vi "setNSteps.vi"(0 "connection ID":refnum<k5>, 1 "axis":i32, 2 "backward":bool, 3 "step":i32, 5 "error in":errorcluster) -> (14 "connection ID":refnum<k5>, 15 "axis_out":i32, 19 "error out":errorcluster)   [LabVIEW 2016]
doc: "This function triggers n steps on the selected axis in desired direction."
panel:
  out "params_cluster":cluster{"axis":i32, "backward":bool, "step":i32}
  in  "Params_cluster":T1
  in  "results_cluster":cluster{"errNo":i32}
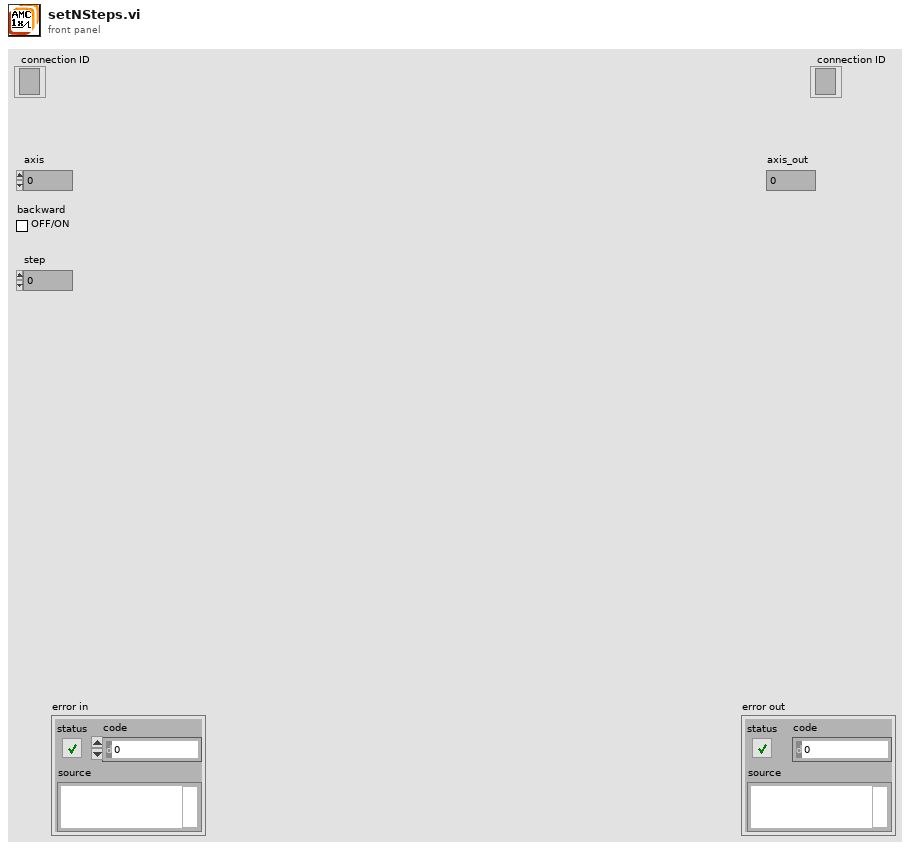
[diagram p1: front panel]
types:
  T1 = cluster{"integer":i32, "boolean":bool, "integer":i32}
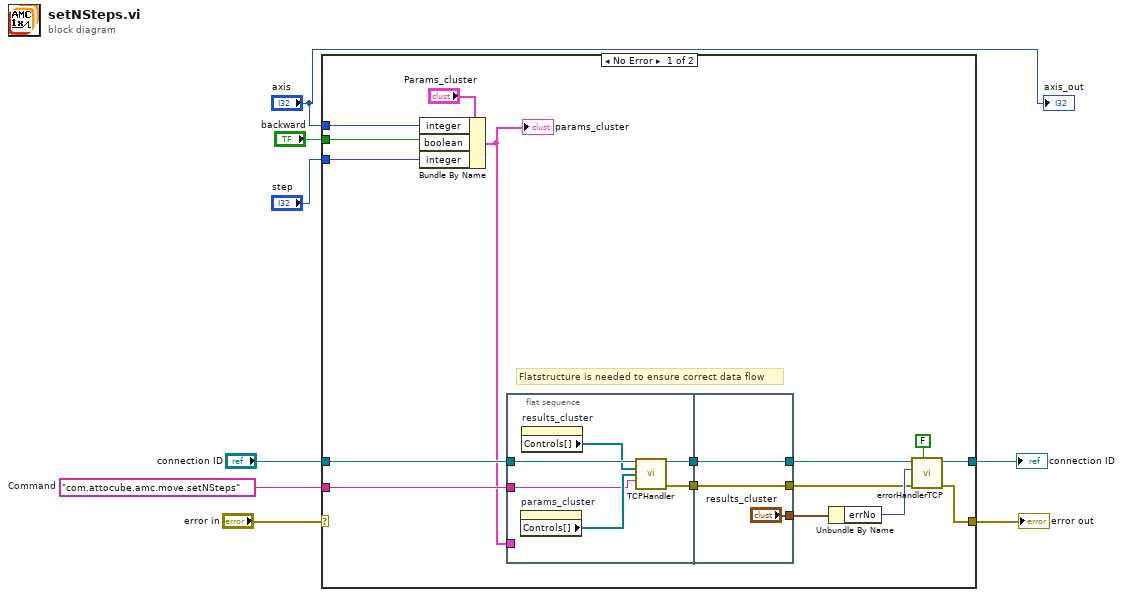
[diagram p0: block diagram]
diagram:
  w4 = "com.attocube.amc.move.setNSteps"  # Command
  n1 = case shown="No Error" "error in" {
    selector: "error in" -> [_ w35]
    tunnel: [w22 w35] -> w8
    tunnel: [w24 w34] -> w7
    tunnel: "connection ID" -> [w21 w34]
    tunnel: w4 -> [w15 _]
    tunnel: "axis" -> [w11 _]
    tunnel: "backward" -> [w10 _]
    tunnel: "step" -> [w9 _]
    frame No Error {
      # "Flatstructure is needed to ensure correct data flow"
      n2 = Bundle By Name(cluster="Params_cluster", "integer"=w11, "boolean"=w10, "integer"=w9) -> (w12:T1)
      "params_cluster" <- w12
      n3 = flat-sequence {
        tunnel: [w29] -> w17
        tunnel: w21 -> [w30]
        tunnel: w15 -> [w26]
        tunnel: [w25] -> w13
        tunnel: w12 -> [_]
        tunnel: ["results_cluster"] -> w18
        tunnel: [w33] -> w20
        tunnel: w17 -> [w33]
        tunnel: [w31] -> w14
        tunnel: w13 -> [w31]
        frame #0 {
          n4 = property on="params_cluster" class="Clust (strict)"() -> ("Controls[]"=w27:refnum<vi>[])  [unwired: 2 in, 2 out]
          n5 = property on="results_cluster" class="Clust (strict)"() -> ("Controls[]"=w28:refnum<vi>[])  [unwired: 2 in, 2 out]
          n6 = call "TCPHandler.vi"("connection ID"=w30, "results_cluster"=w28, "params_cluster"=w27, "method"=w26) -> ("connection ID"=w29:refnum<k5>, "error"=w25:errorcluster)  [unwired: 8 in, 2 out]
        }
        frame #1 {
        }
      }
      n7 = Unbundle By Name(w18) -> ("errNo"=w19:i32)
      n8 = call "errorHandlerTCP.vi"("show popup"=FALSE, "error in"=w14, "error number"=w19, "connection ID"=w20) -> ("error out"=w22:errorcluster, "connection ID"=w24:refnum<k5>)  [unwired: 6 in]
    }
    frame Error {
    }
  }
  "error out" <- w8
  "connection ID" <- w7
  "axis_out" <- "axis"
